vi "convert_voltage_to_opening.vi"(8 "status_in":bool, 10 "bypass_valve_voltage":dbl, 11 "run_valve_voltage":dbl) -> (0 "status_out":bool, 2 "bypass_valve_opening":dbl, 3 "run_valve_opening":dbl)   [LabVIEW 2019]
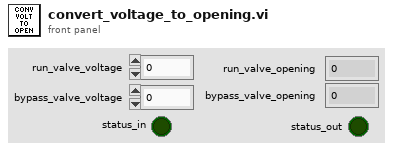
[diagram p1: front panel]
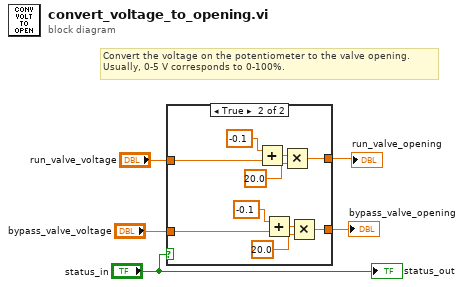
[diagram p0: block diagram]
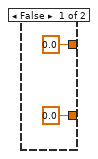
[diagram p2: hidden frame]
diagram:
  # "Convert the voltage on the potentiometer to the valve opening.\nUsually, 0-5 V corresponds to 0-100%."
  n1 = case shown="True" "status_in" {
    tunnel: [0.0 w11] -> w5
    tunnel: [0.0 w10] -> w4
    tunnel: "run_valve_voltage" -> [_ w9]
    tunnel: "bypass_valve_voltage" -> [_ w8]
    frame False {
    }
    frame True {
      n2 = Add(x=-0.1, y=w9) -> (x+y=w17:dbl)
      n3 = Add(x=-0.1, y=w8) -> (x+y=w14:dbl)
      n4 = Multiply(x=w17, y=20.0) -> (x*y=w11:dbl)
      n5 = Multiply(x=w14, y=20.0) -> (x*y=w10:dbl)
    }
  }
  "run_valve_opening" <- w5
  "bypass_valve_opening" <- w4
  "status_out" <- "status_in"
